vi "BME_DG_SetCalibrationLevel.vi"(7 "error in (no error)":errorcluster, 9 "CalibrationLevel":T1(ring)=enum."CalibrateIncrement", 10 "DG_Number":i32) -> (0 "error out":errorcluster, 3 "return code":i32)   [LabVIEW 2009]
uses:
  BME Beispiele/BME DLL/DelayGenerator.dll
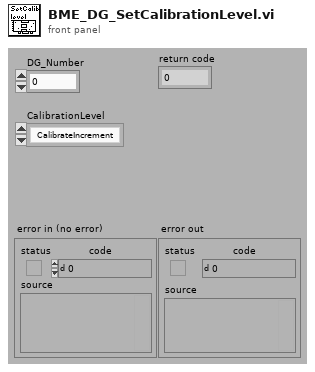
[diagram p1: front panel]
types:
  T1 = enum16{"NoCalibration", "CalibrateIncrement", "CalibrateOffset"}
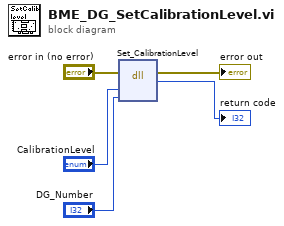
[diagram p0: block diagram]
diagram:
  n1 = dll-call lib="C:/Dokumente und Einstellungen/A2.5/Desktop/BME Beispiele/BME DLL/DelayGenerator.dll" fn="Set_CalibrationLevel" label="Initialize_DG_BME"(error in="error in (no error)", "CalibrationLevel"="CalibrationLevel", "DG_Number"="DG_Number") -> (error out=→"error out":errorcluster, "return type"=→"return code":i32)  [unwired: 4 in, 1 out]
